vi "Launcher.vi"() -> ()   [LabVIEW 2020]
uses:
  <vilib>/ActorFramework/Message Enqueuer/Message Enqueuer.lvclass
  Contador/Contador.lvclass
  C:/Program Files (x86)/National Instruments/LabVIEW 2020/vi.lib/ActorFramework/Actor/Actor.lvclass
  <vilib>/ActorFramework/Message Enqueuer/Message Enqueuer.lvclass/Message Enqueuer.ctl
  <vilib>/ActorFramework/Message Enqueuer/Enqueue.vi
  <vilib>/ActorFramework/Stop Msg/Stop Msg.lvclass
  C:/Program Files (x86)/National Instruments/LabVIEW 2020/vi.lib/ActorFramework/Message/Message.lvclass
  <vilib>/ActorFramework/Message Priority Queue/Priority Enqueue.vi
  <vilib>/ActorFramework/Actor/Actor.lvclass
panel:
  in  "Exit":bool
  in  "stop":bool
  in  "Counter":u16(ring)
  in  "Add Button":bool
  in  "Type":enum16{"Generador", "Binario"}(ring)
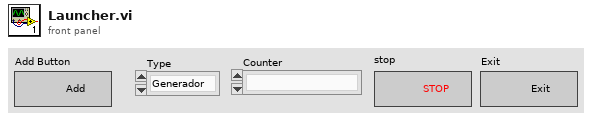
[diagram p1: front panel]
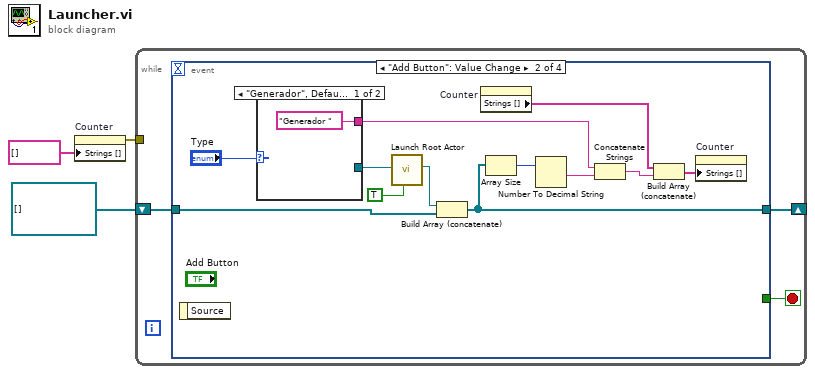
[diagram p0: block diagram]
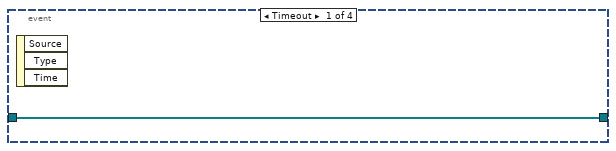
[diagram p2: hidden frame]
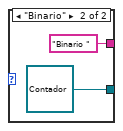
[diagram p3: hidden frame]
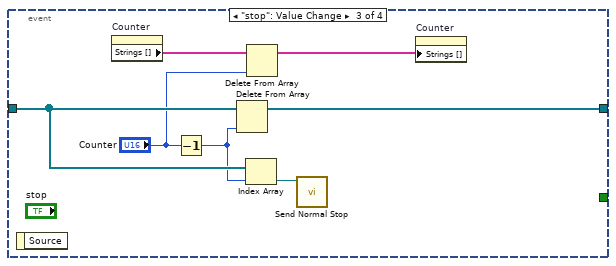
[diagram p4: hidden frame]
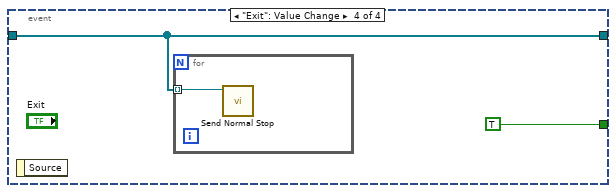
[diagram p5: hidden frame]
diagram:
  n1 = property on="Counter" class="Ring (strict)"("Strings []"=string[] []) -> (error out=w2:errorcluster)  [unwired: 2 in, 1 out]
  n2 = while {
    tunnel: w2 -> [_]
    shift-right: [w5] -> _
    shift-left: refnum<class "Message Enqueuer.lvclass">[] [] -> [w6]
    stop <- w4 stop-if-true
    n3 = event shown="[1] \"Add Button\": Value Change" {
      selector: _ -> [_ _ _ _]
      dyn-events: _ -> [_ _ _ _]
      timeout: _ -> [_ _ _ _]
      tunnel: w6 -> [w7 w15 w29 w30]
      tunnel: [w7 w13 w27 w30] -> w5
      tunnel: [_ _ _ TRUE] -> w4
      event Timeout {
        n4 = event-data() -> ()  [unwired: 1 in, 3 out]
      }
      event "Add Button": Value Change {
        n5 = event-data() -> ()  [unwired: 1 in, 1 out]
        n6 = case shown="\"Generador\", Default" "Type" {
          tunnel: [_ refnum<class "Contador.lvclass"> refnum ("Contador.lvlib:Contador.lvclass")] -> w14
          tunnel: ["Generador " ("string") "Binario " ("string")] -> w8
          frame "Generador", Default {
          }
          frame "Binario" {
          }
        }
        n7 = call <vilib>:"Launch Root Actor.vi"("Open Actor Core front panel? (F)"=TRUE, "Actor"=w14) -> ("Actor's Enqueuer"=w17:refnum<class "Message Enqueuer.lvclass">)  [unwired: 8 in, 1 out]
        n8 = Build Array (concatenate) "Build Array"(w17, w15) -> (w13:refnum<class "Message Enqueuer.lvclass">[])
        n9 = property on="Counter" class="Ring (strict)"() -> ("Strings []"=w11:string[])  [unwired: 2 in, 2 out]
        n10 = Array Size(array=w13) -> (size(s)=w18:i32)
        n11 = Number To Decimal String(number=w18) -> (decimal integer string=w19:string)  [unwired: 1 in]
        n12 = Concatenate Strings(w8, w19) -> (w9:string)
        n13 = Build Array (concatenate) "Build Array"(w11, w9) -> (w16:string[])
        n14 = property on="Counter" class="Ring (strict)"("Strings []"=w16) -> ()  [unwired: 2 in, 2 out]
      }
      event "stop": Value Change {
        n15 = event-data() -> ()  [unwired: 1 in, 1 out]
        n16 = property on="Counter" class="Ring (strict)"() -> ("Strings []"=w26:string[])  [unwired: 2 in, 2 out]
        n17 = Decrement(x="Counter") -> (x-1=w24:u16)
        n18 = Delete From Array(array=w29, index=w24) -> (array with subset deleted=w27:refnum<class "Message Enqueuer.lvclass">[])  [unwired: 1 in, 1 out]
        n19 = Index Array "Index Array"(array=w29, index=w24) -> (element=w28:refnum<class "Message Enqueuer.lvclass">)
        n20 = Delete From Array(array=w26, index="Counter") -> (array with subset deleted=w25:string[])  [unwired: 1 in, 1 out]
        n21 = call <vilib>:"Send Normal Stop.vi"("Message Enqueuer"=w28) -> ()  [unwired: 10 in, 1 out]
        n22 = property on="Counter" class="Ring (strict)"("Strings []"=w25) -> ()  [unwired: 2 in, 2 out]
      }
      event "Exit": Value Change {
        n23 = event-data() -> ()  [unwired: 1 in, 1 out]
        n24 = for {
          tunnel: w30 -> [w32] mode=indexing
          n25 = call <vilib>:"Send Normal Stop.vi"("Message Enqueuer"=w32) -> ()  [unwired: 10 in, 1 out]
        }
      }
    }
  }
